vi "Snapshot test.vi"() -> ()   [LabVIEW 2016]
uses:
  Q:/Common/DLLs/GEA3/GeaCommunication.dll
  Common/DLLs/GEA3/GeaCommunication.dll
  Common/LabVIEW GEA2 Toolkit/LabVIEW_GEA2_Toolkit.lvlibp/type defs/Source_Destination.ctl
  Common/LabVIEW GEA2 Toolkit/LabVIEW_GEA2_Toolkit.lvlibp
panel:
  in  "Standalone":bool
  out "Output Snap Data":T1(array[cluster])
  out "Error Out":errorcluster
  out "GEA2 Reference Out":refnum<k24>
  in  "Error In":errorcluster
  in  "GEA Inputs":T2={"Source"=228, "Destination"=35} {"Destination" format="%.0x"; "Source" format="%.0x"}
  in  "GEA2 Reference In":refnum<k24>
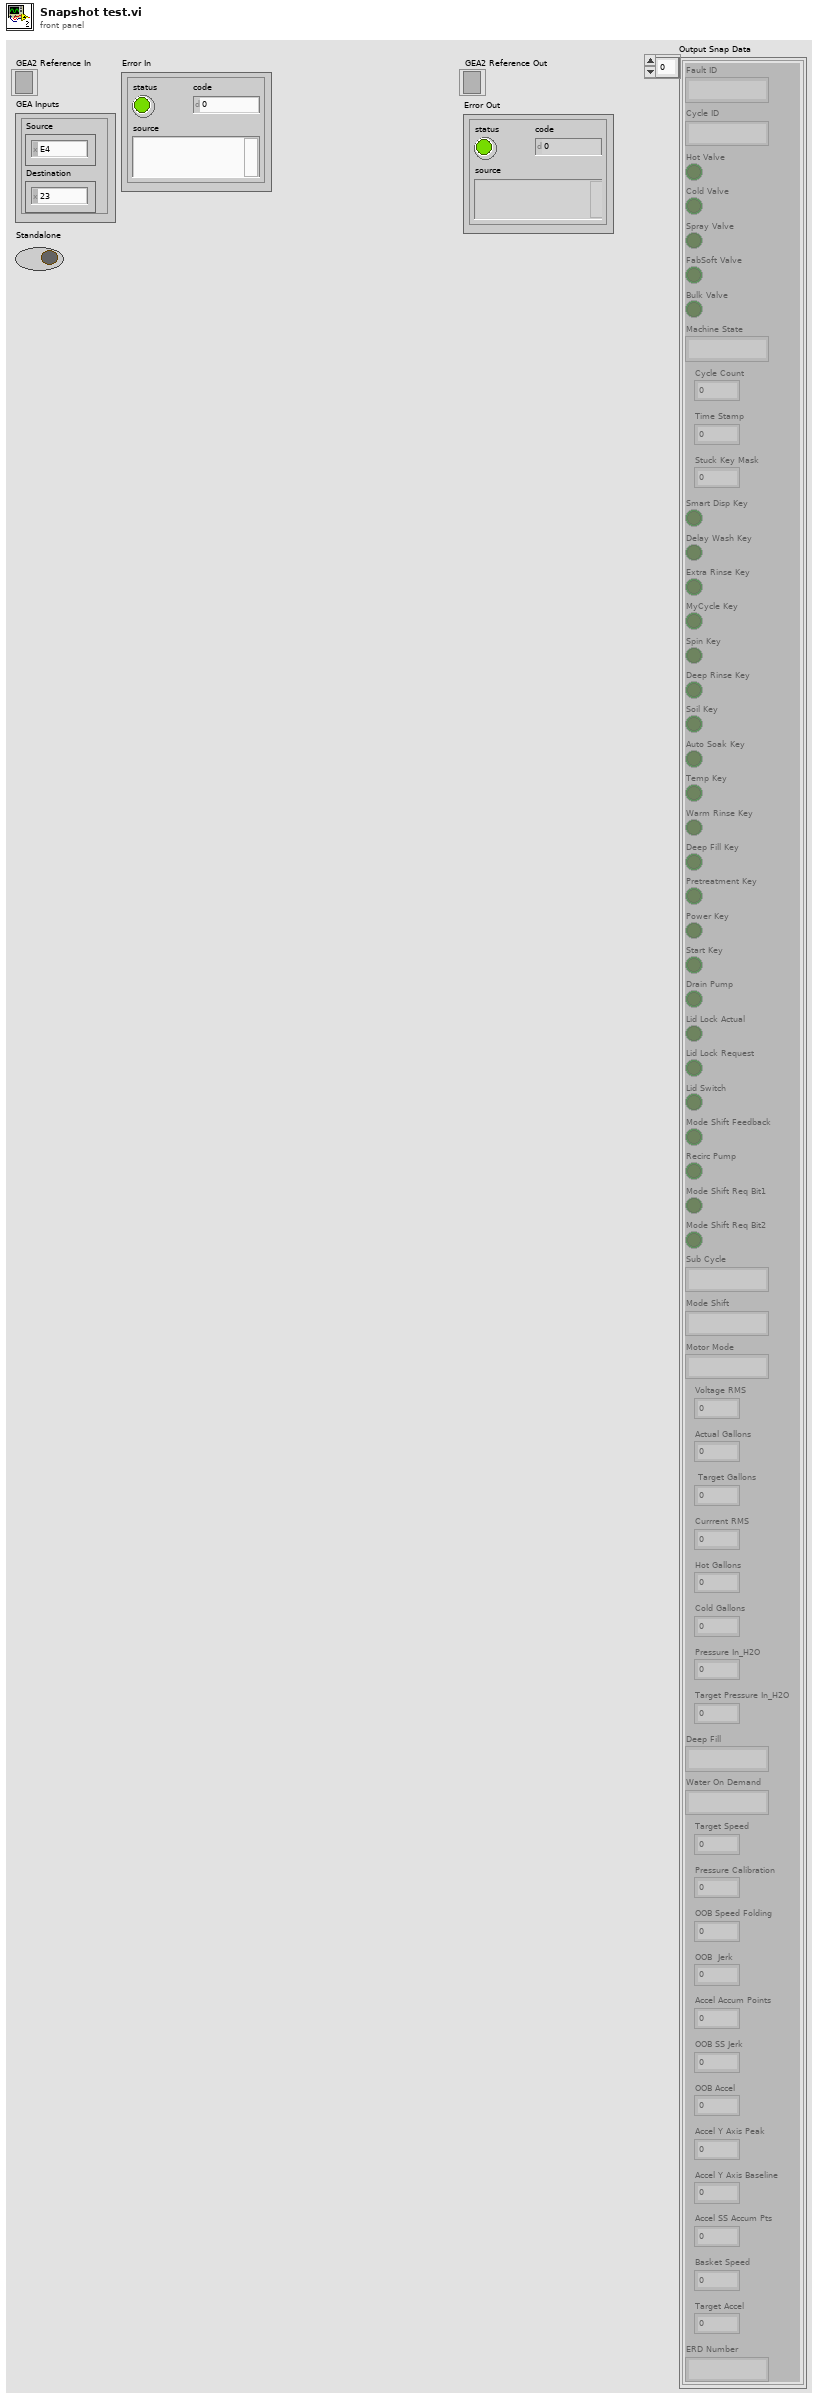
[diagram p1: front panel]
types:
  T1 = cluster{"Fault ID":string, "Cycle ID":string, "Hot Valve":bool, "Cold Valve":bool, "Spray Valve":bool, "FabSoft Valve":bool, "Bulk Valve":bool, "Machine State":string, "Cycle Count":u32, "Time Stamp":u32, "Stuck Key Mask ":u64, "Smart Disp Key":bool, "Delay Wash Key":bool, "Extra Rinse Key":bool, "MyCycle Key":bool, "Spin Key":bool, "Deep Rinse Key":bool, "Soil Key":bool, "Auto Soak Key":bool, "Temp Key":bool, "Warm Rinse Key":bool, "Deep Fill Key":bool, "Pretreatment Key":bool, "Power Key":bool, "Start Key":bool, "Drain Pump":bool, "Lid Lock Actual":bool, "Lid Lock Request":bool, "Lid Switch":bool, "Mode Shift Feedback":bool, "Recirc Pump":bool, "Mode Shift Req Bit1":bool, "Mode Shift Req Bit2":bool, "Sub Cycle":string, "Mode Shift":string, "Motor Mode":string, "Voltage RMS":u16, "Actual Gallons":u16, " Target Gallons":u16, "Currrent RMS":u16, "Hot Gallons":u16, "Cold Gallons":u16, "Pressure In_H2O":u32, "Target Pressure In_H2O":dbl, "Deep Fill":string, "Water On Demand":string, "Target Speed":i16, "Pressure Calibration":u32, "OOB Speed Folding":i32, "OOB  Jerk":i32, "Accel Accum Points":u8, "OOB SS Jerk":i32, "OOB Accel":i32, "Accel Y Axis Peak":i16, "Accel Y Axis Baseline":i16, "Accel SS Accum Pts":u8, "Basket Speed":u16, "Target Accel":u16, "ERD Number":string}[]
  T2 = typedef "LabVIEW_GEA2_Toolkit.lvlibp/Source_Destination.ctl" = cluster{"Source":u8, "Destination":u8}
  T3 = cluster{"Fault ID":u16, "Cycle ID":u8, "Cycle Count":u32, "Time Stamp":u32, "Water Valve":u8, "Stuck Key Mask":u64, "Pump-Lid-Mode":u8, "Machine State":u8, "Sub Cycle":u8, "Mode Shift":u8, "Motor Mode":u8, "Target Speed":i16, "Voltage RMS":u16, "Actual Gallons":u16, "Target Accel":u16, "Current RMS":u16, "Target Gallons":u16, "Hot Gallons":u16, "Pressure Cal":u32, "Cold Gallons":u16, "Pressure ":u32, "Target Pressure":u32, "OOB Folding":i32, "Acel SS Pts":u8, "OOB Jerk":i32, "Deep Fill":u8, "Water On Demand":u8, "OOB Accel":i32, "Acel Accum Pts":u8, "Acel Y Axis Base":i16, "Acel Y Axis PK":i16, "Unused":u8, "Basket Speed":u16, "OOB SS Jerk":i32, "ERD Number":u64}[]
  T4 = typedef "Control 6.ctl" = cluster{"Fault ID":string, "Cycle ID":string, "Hot Valve":bool, "Cold Valve":bool, "Spray Valve":bool, "FabSoft Valve":bool, "Bulk Valve":bool, "Machine State":string, "Cycle Count":u32, "Time Stamp":u32, "Stuck Key Mask ":u64, "Smart Disp Key":bool, "Delay Wash Key":bool, "Extra Rinse Key":bool, "MyCycle Key":bool, "Spin Key":bool, "Deep Rinse Key":bool, "Soil Key":bool, "Auto Soak Key":bool, "Temp Key":bool, "Warm Rinse Key":bool, "Deep Fill Key":bool, "Pretreatment Key":bool, "Power Key":bool, "Start Key":bool, "Drain Pump":bool, "Lid Lock Actual":bool, "Lid Lock Request":bool, "Lid Switch":bool, "Mode Shift Feedback":bool, "Recirc Pump":bool, "Mode Shift Req Bit1":bool, "Mode Shift Req Bit2":bool, "Sub Cycle":string, "Mode Shift":string, "Motor Mode":string, "Voltage RMS":u16, "Actual Gallons":u16, " Target Gallons":u16, "Currrent RMS":u16, "Hot Gallons":u16, "Cold Gallons":u16, "Pressure In_H2O":u32, "Target Pressure In_H2O":dbl, "Deep Fill":string, "Water On Demand":string, "Target Speed":i16, "Pressure Calibration":u32, "OOB Speed Folding":i32, "OOB  Jerk":i32, "Accel Accum Points":u8, "OOB SS Jerk":i32, "OOB Accel":i32, "Accel Y Axis Peak":i16, "Accel Y Axis Baseline":i16, "Accel SS Accum Pts":u8, "Basket Speed":u16, "Target Accel":u16, "ERD Number":string}
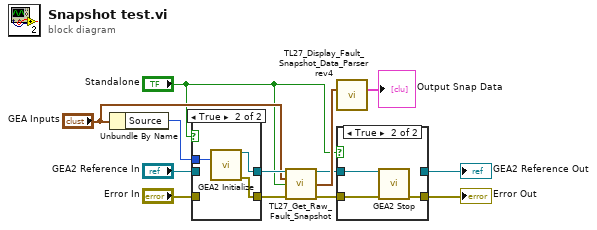
[diagram p0: block diagram]
diagram:
  n1 = Unbundle By Name("GEA Inputs") -> ("Source"=w10:u8)
  n2 = case shown="True" "Standalone" {
    tunnel: [w15 w17] -> w6
    tunnel: "Error In" -> [w15 _]
    tunnel: [w14 w18] -> w8
    tunnel: "GEA2 Reference In" -> [w14 _]
    tunnel: w10 -> [_ w16]
    frame False {
    }
    frame True {
      n3 = call "GEA2 Initialize.vi"("Source Address"=w16) -> ("GEA2 Reference Out"=w18:refnum<k24>, "error out"=w17:errorcluster)  [unwired: 12 in, 1 out]
    }
  }
  n4 = call "TL27_Get_Raw_Fault_Snapshot.vi"("GEA2 Reference In"=w8, "GEA Inputs"="GEA Inputs", "Standalone"="Standalone", "Error In"=w6) -> ("GEA2 Reference Out"=w3:refnum<k24>, "Array"=w13:T3, "Error Out"=w2:errorcluster)  [unwired: 9 in]
  n5 = call "TL27_Display_Fault_Snapshot_Data_Parser rev4.vi"("Input Snao Data"=w13) -> ("Output Snap Data"=→"Output Snap Data":T4[])  [unwired: 14 in]
  n6 = case shown="True" "Standalone" {
    tunnel: w3 -> [w20 w23]
    tunnel: [w20 _] -> w5
    tunnel: w2 -> [w19 w22]
    tunnel: [w19 w21] -> w4
    frame False {
    }
    frame True {
      n7 = call "GEA2 Stop.vi"("GEA2 Reference In"=w23, "Error In"=w22) -> ("Error Out"=w21:errorcluster)  [unwired: 13 in]
    }
  }
  "GEA2 Reference Out" <- w5
  "Error Out" <- w4
